vi "NI_Security Globals.vi"() -> ()   [LabVIEW 2020]
panel:
  in  "machine/domain separator":string="::"
  in  "domain/principal separator":string="\\"
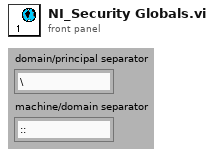
[diagram p1: front panel]
diagram:
